vi "单例模式DEMO(Sender).vi"() -> ()   [LabVIEW 2013]
uses:
  Single_class/Single.lvclass
panel:
  in  "停止":bool
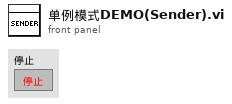
[diagram p1: front panel]
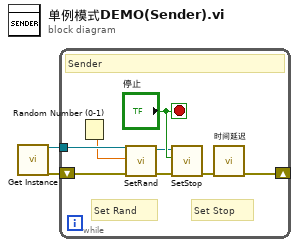
[diagram p0: block diagram]
diagram:
  n1 = call "Get Instance.vi"() -> ("reference out"=w1:refnum<class "Single.lvclass">, "error out"=w2:errorcluster)  [unwired: 18 in]
  n2 = while {
    shift-right: [w3] -> _
    shift-left: w2 -> [w9]
    tunnel: w1 -> [w10]
    stop <- "停止" stop-if-true
    # "Set Stop"
    # "Set Rand"
    # "Sender"
    n3 = Random Number (0-1)() -> (number: 0 to 1=w8:dbl)
    n4 = call "SetRand.vi"("error in (no error)"=w9, "Rand"=w8, "reference in"=w10) -> ("error out"=w7:errorcluster, "reference out"=w4:refnum<class "Single.lvclass">)  [unwired: 7 in]
    n5 = call-dynamic "SetStop.vi"("error in (no error)"=w7, "Stop"="停止", "reference in"=w4) -> ("error out"=w6:errorcluster)  [unwired: 7 in, 1 out]
    n6 = call "时间延迟"("error in (no error)"=w6) -> ("error out"=w3:errorcluster)  [unwired: 10 in]
  }
